vi "SVL Scale Voltage to EU (N Ch - 1 Info).vi"(7 "write waveform attributes? (T)":bool=TRUE, 8 "error in (no error)":errorcluster, 10 "channel info":T1={"sensor sensitivity"=1000.0, "engineering units"=1, "dB reference"=1.0, "custom label"="EU", "weighting filter"=0, "pregain"=0.0} {"pregain" format="%.2f"; "weighting filter" items=["Linear", "A-weighting", "B-weighting", "C-weighting", "ITU-R 468-4", "Dolby", "CCITT", "C-message", "Wb", "Wc", "Wd", "We", "Wf", "Wh", "Wj", "Wk", "Wm", "AES17 20 kHz lowpass", "AES17 40 kHz lowpass", "AES17 20 kHz highpass", "AES17 40 kHz highpass"]; "dB reference" format="%^.1e"; "engineering units" items=["custom..."=0, "V"=1, "A"=21, "C"=30, "pC"=31, "s"=32, "-"=29, "Pa"=2, "N"=20, "g"=3, "m/s^2"=4, "m/s"=5, "m"=6, "mm/s"=12, "mm"=13, "micron/s"=14, "micron"=15, "in/s^2"=7, "in/s"=8, "in"=9, "mil/s"=10, "mil"=11, "rad/s^2"=16, "rad/s"=17, "rad"=18, "deg/s^2"=26, "deg/s"=27, "deg"=28, "RPM"=22, "cycle/s^2"=23, "Hz"=24, "cycle"=25, "strain"=19]; "sensor sensitivity" format="%#_5f"}, 11 "signals [V]":waveform(dbl)[](array[waveform])=[{"t0"=timestamp(0 s since 1904-01-01), "dt"=1.0, "Y"=[]}]) -> (0 "error out":errorcluster, 2 "unit label":string, 3 "scaled signals [EU]":waveform(dbl)[](array[waveform]))   [LabVIEW 2017, in "SoundVib_Calibration.lvlib"]
doc: "Scales <B>signal [V]</B> from volts to the engineering units (EU) you select. Wire data to the <B>signal [V]</B> input to determine the polymorphic instance to use or manually select the instance."
uses:
  <vilib>/addons/Sound and Vibration/svt_Calibration/SoundVib_Calibration.lvlib
  <vilib>/addons/_NISVFA/_Shared subVIs/Controls/svc_Channel Info.ctl
  <vilib>/addons/_NISVFA/_Shared subVIs/Controls/svc_Engineering Units Text Ring.ctl
  <vilib>/addons/_NISVFA/_Shared subVIs/Controls/svc_Weighting Filter Text Ring.ctl
  <vilib>/addons/_NISVFA/_Shared subVIs/Common/svc_Set SV Channel Info.vi
  <vilib>/addons/_NISVFA/_Shared subVIs/Common/svc_Set SV Channel Info (variant).vi
  <vilib>/addons/_NISVFA/_Shared subVIs/Common/SVL Set dB Reference (variant).vi
  <vilib>/addons/_NISVFA/_Shared subVIs/Common/svc_Engineering Units to Unit Label.vi
  <vilib>/addons/_NISVFA/_Shared subVIs/Common/svc_Set dB ref if Pascal.vi
  <vilib>/addons/_NISVFA/_Shared subVIs/Common/svc_Compute Scale Factor to Convert C to EU.vi
  <vilib>/addons/_NISVFA/_Shared subVIs/Common/svc_Compute Scale Factor to Convert V to EU.vi
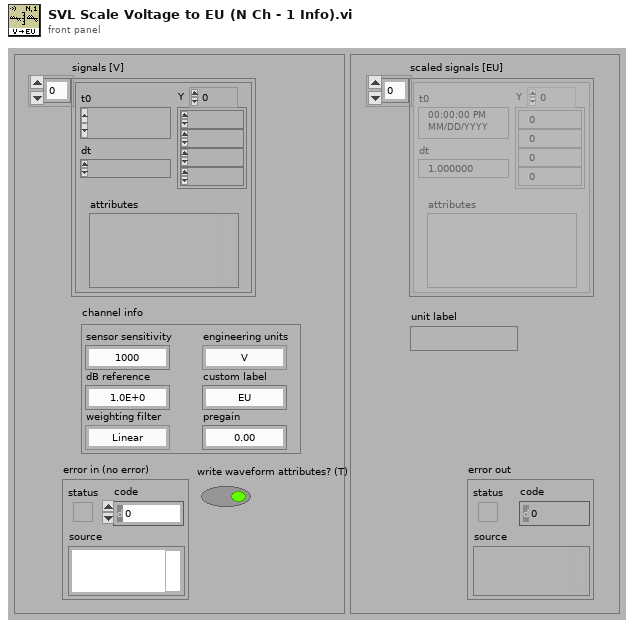
[diagram p1: front panel]
types:
  T1 = typedef "svc_Channel Info.ctl" = cluster{"sensor sensitivity":dbl, "engineering units":T2, "dB reference":dbl, "custom label":string, "weighting filter":T3, "pregain":dbl}
  T2 = typedef "svc_Engineering Units Text Ring.ctl" = u16
  T3 = typedef "svc_Weighting Filter Text Ring.ctl" = u16
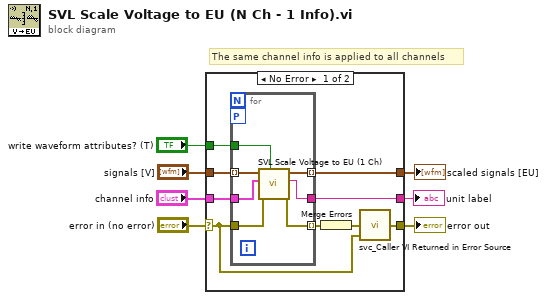
[diagram p0: block diagram]
diagram:
  # "The same channel info is applied to all channels"
  n1 = case shown="No Error" "error in (no error)" {
    selector: "error in (no error)" -> [w10 w24]
    tunnel: "signals [V]" -> [w16 _]
    tunnel: "channel info" -> [w15 _]
    tunnel: [w14 _] -> w6
    tunnel: [w11 w24] -> w5
    tunnel: [w13 _] -> w3
    tunnel: "write waveform attributes? (T)" -> [w9 _]
    frame No Error {
      n2 = for {
        tunnel: w16 -> [w23] mode=indexing
        tunnel: w15 -> [w22]
        tunnel: [w21] -> w14 mode=indexing
        tunnel: [w20] -> w13
        tunnel: w9 -> [w19]
        workers-P: _ -> [_]
        tunnel: w10 -> [w18]
        tunnel: [w17] -> w12 mode=indexing
        n3 = call <vilib>:"SVL Scale Voltage to EU (1 Ch).vi"("write waveform attributes? (T)"=w19, "error in (no error)"=w18, "channel info"=w22, "signal [V]"=w23) -> ("error out"=w17:errorcluster, "unit label"=w20:string, "scaled signal [EU]"=w21:waveform(dbl))  [unwired: 5 in]
      }
      n4 = Merge Errors(w12) -> (w8:errorcluster)
      n5 = call <vilib>:"svc_Caller VI Returned in Error Source.vi"("warning input to caller"=w10, "error in (no error)"=w8) -> ("error out"=w11:errorcluster)  [unwired: 3 in]
    }
    frame Error {
    }
  }
  "scaled signals [EU]" <- w6
  "error out" <- w5
  "unit label" <- w3
